vi "gfitsio-write-image-vi-data.vi"(7 "requested data":T1(ring)=enum."diagram, panel, .vi file", 8 "error in (no error)":errorcluster, 9 "vi depth (1)":i32=1, 11 "gfits refnum":T2=refnum) -> (0 "error out":errorcluster, 3 "dup gfits refnum":T2)   [LabVIEW 2013]
uses:
  gfitsio-refnum.ctl
  cfitsio-bitpix.ctl
  gfitsio-write-image-subset-variant.vi
  gfitsio-write-image-subset-u8-1d.vi
  gfitsio.lvlib
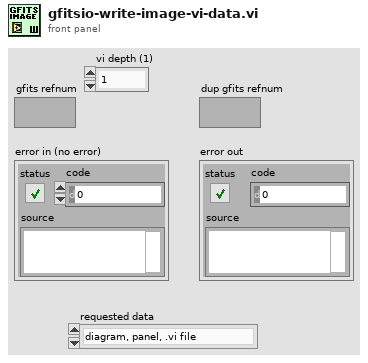
[diagram p1: front panel]
types:
  T1 = enum16{"diagram", "panel", ".vi file", "diagram, panel", "diagram, .vi file", "panel, .vi file", "diagram, panel, .vi file"}
  T2 = typedef "gfitsio.lvlib/gfitsio-refnum.ctl" = refnum<k1>
  T3 = typedef "gfitsio.lvlib/cfitsio-bitpix.ctl" = i32
  T4 = typedef "imagedata.ctl" = cluster{"image type":i32, "image depth":i32, "image":u8[], "mask":u8[], "colors":u32[], "Rectangle":cluster{"left":i16, "top":i16, "right":i16, "bottom":i16}}
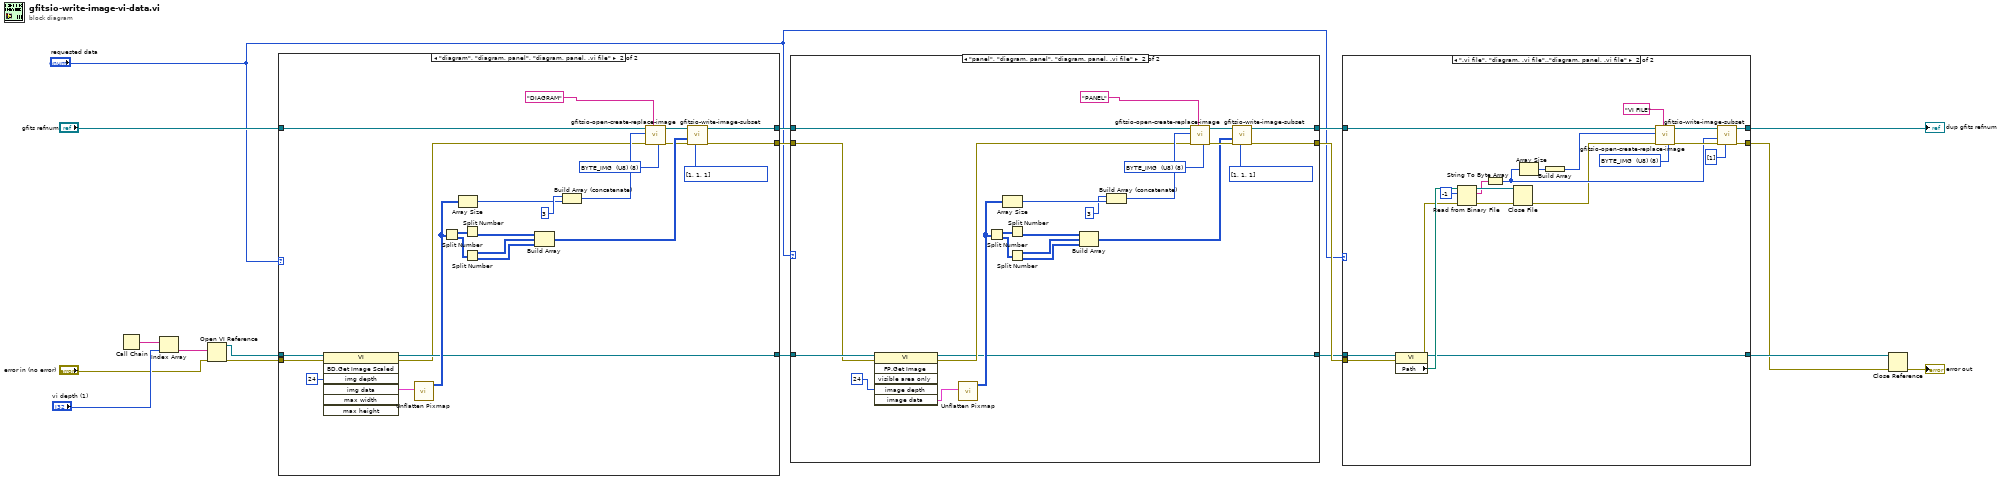
[diagram p0: block diagram]
diagram:
  n1 = Call Chain() -> (call chain=w17:string[])
  n2 = Index Array(array=w17, index="vi depth (1)") -> (element=w14:string)
  n3 = Open VI Reference(vi path=w14, error in (no error)="error in (no error)") -> (vi reference=w13:refnum<vi>, error out=w12:errorcluster)  [unwired: 4 in]
  n4 = case shown="\"diagram\", \"diagram, panel\", \"diagram, panel, .vi file\"" "requested data" {
    tunnel: "gfits refnum" -> [w19 w31]
    tunnel: w12 -> [w20 w28]
    tunnel: w13 -> [w21 w27]
    tunnel: [w19 w26] -> w10
    tunnel: [w21 w24] -> w9
    tunnel: [w20 w22] -> w8
    frame Default {
    }
    frame "diagram", "diagram, panel", "diagram, panel, .vi file" {
      w33 = T3 8 items=["<invalid type>"=0, "BYTE_IMG  (U8)"=8, "SHORT_IMG  (I16)"=16, "USHORT_IMG  (U16)"=20, "LONG_IMG  (I32)"=32, "ULONG_IMG  (U32)"=40, "FLOAT_IMG  (SGL)"=-32, "DOUBLE_IMG  (DBL)"=-64] ("image data type")
      n5 = invoke class="VI" method="BD.Get Image Scaled"(reference=w27, error in=w28, "img depth"=24 ("Image Depth")) -> (reference out=w24:refnum<vi>, error out=w23:errorcluster, "img data"=w29:T4)  [unwired: 4 in, 4 out]
      n6 = call <vilib>:"Unflatten Pixmap.vi"("image data"=w29) -> ("24-bit pixmap"=w36:u32[][])  [unwired: 4 in, 6 out]
      n7 = Split Number(x=w36) -> (hi(x)=w34:u16[][], lo(x)=w35:u16[][])
      n8 = Array Size(array=w36) -> (size(s)=w32:i32[])
      n9 = Split Number(x=w34) -> (lo(x)=w43:u8[][])  [unwired: 1 out]
      n10 = Split Number(x=w35) -> (hi(x)=w44:u8[][], lo(x)=w45:u8[][])
      n11 = Build Array(w43, w44, w45) -> (w42:u8[][][])
      n12 = Build Array (concatenate)(3, w32) -> (w40:i32[])
      n13 = call "gfitsio-open-create-replace-image.vi"("image data type"=w33, "hdu name (dialog if empty)"="DIAGRAM", "error in (no error)"=w23, "naxes"=w40, "gfits refnum"=w31) -> ("error out"=w37:errorcluster, "dup gfits refnum"=w38:T2)  [unwired: 4 in, 1 out]
      n14 = call-poly "gfitsio-write-image-subset.vi"("fpixel"=i32[] [1, 1, 1] ("size(s)"), "error in (no error)"=w37, "data"=w42, "gfits refnum"=w38) -> ("error out"=w22:errorcluster, "dup gfits refnum"=w26:T2)  [unwired: 6 in]
    }
  }
  n15 = case shown="\"panel\", \"diagram, panel\", \"diagram, panel, .vi file\"" "requested data" {
    tunnel: w10 -> [w48 w58]
    tunnel: w9 -> [w46 w56]
    tunnel: w8 -> [w47 w55]
    tunnel: [w47 w53] -> w7
    tunnel: [w46 w52] -> w6
    tunnel: [w48 w51] -> w2
    frame Default {
    }
    frame "panel", "diagram, panel", "diagram, panel, .vi file" {
      w71 = T3 8 items=["<invalid type>"=0, "BYTE_IMG  (U8)"=8, "SHORT_IMG  (I16)"=16, "USHORT_IMG  (U16)"=20, "LONG_IMG  (I32)"=32, "ULONG_IMG  (U32)"=40, "FLOAT_IMG  (SGL)"=-32, "DOUBLE_IMG  (DBL)"=-64] ("image data type")
      n16 = invoke class="VI" method="FP.Get Image"(reference=w56, error in=w55, "image depth"=24 ("Image Depth")) -> (reference out=w52:refnum<vi>, error out=w54:errorcluster, "image data"=w49:T4)  [unwired: 3 in, 3 out]
      n17 = call <vilib>:"Unflatten Pixmap.vi"("image data"=w49) -> ("24-bit pixmap"=w68:u32[][])  [unwired: 4 in, 6 out]
      n18 = Split Number(x=w68) -> (hi(x)=w70:u16[][], lo(x)=w69:u16[][])
      n19 = Array Size(array=w68) -> (size(s)=w72:i32[])
      n20 = Split Number(x=w70) -> (lo(x)=w61:u8[][])  [unwired: 1 out]
      n21 = Split Number(x=w69) -> (hi(x)=w60:u8[][], lo(x)=w59:u8[][])
      n22 = Build Array(w61, w60, w59) -> (w62:u8[][][])
      n23 = Build Array (concatenate)(3, w72) -> (w64:i32[])
      n24 = call "gfitsio-open-create-replace-image.vi"("image data type"=w71, "hdu name (dialog if empty)"="PANEL", "error in (no error)"=w54, "naxes"=w64, "gfits refnum"=w58) -> ("error out"=w67:errorcluster, "dup gfits refnum"=w66:T2)  [unwired: 4 in, 1 out]
      n25 = call-poly "gfitsio-write-image-subset.vi"("fpixel"=i32[] [1, 1, 1] ("size(s)"), "error in (no error)"=w67, "data"=w62, "gfits refnum"=w66) -> ("error out"=w53:errorcluster, "dup gfits refnum"=w51:T2)  [unwired: 6 in]
    }
  }
  n26 = case shown="\".vi file\", \"diagram, .vi file\"..\"diagram, panel, .vi file\"" "requested data" {
    tunnel: [w75 w83] -> w11
    tunnel: w7 -> [w74 w82]
    tunnel: w6 -> [w73 w79]
    tunnel: [w73 w78] -> w5
    tunnel: [w74 w77] -> w4
    tunnel: w2 -> [w75 w76]
    frame Default {
    }
    frame ".vi file", "diagram, .vi file".."diagram, panel, .vi file" {
      w87 = T3 8 items=["<invalid type>"=0, "BYTE_IMG  (U8)"=8, "SHORT_IMG  (I16)"=16, "USHORT_IMG  (U16)"=20, "LONG_IMG  (I32)"=32, "ULONG_IMG  (U32)"=40, "FLOAT_IMG  (SGL)"=-32, "DOUBLE_IMG  (DBL)"=-64] ("image data type")
      n27 = property class="VI"(reference=w79, error in=w82) -> (reference out=w78:refnum<vi>, error out=w81:errorcluster, "Path"=w85:path)
      n28 = Read from Binary File(8:w81, 10:-1 ("count (1)"), 11:w85) -> (0:w96:errorcluster, 2:w94:string, 3:w95:refnum<file>)  [unwired: 3 in, 1 out]
      n29 = String To Byte Array(string=w94) -> (unsigned byte array=w90:u8[])
      n30 = Close File(refnum=w95, error in=w96) -> (error out=w80:errorcluster)  [unwired: 1 out]
      n31 = Array Size(array=w90) -> (size(s)=w89:i32)
      n32 = Build Array(w89) -> (w88:i32[])
      n33 = call "gfitsio-open-create-replace-image.vi"("image data type"=w87, "hdu name (dialog if empty)"="VI FILE", "error in (no error)"=w80, "naxes"=w88, "gfits refnum"=w76) -> ("error out"=w92:errorcluster, "dup gfits refnum"=w93:T2)  [unwired: 4 in, 1 out]
      n34 = call-poly "gfitsio-write-image-subset.vi"("fpixel"=i32[] [1], "error in (no error)"=w92, "data"=w90, "gfits refnum"=w93) -> ("error out"=w77:errorcluster, "dup gfits refnum"=w83:T2)  [unwired: 6 in]
    }
  }
  "dup gfits refnum" <- w11
  n35 = Close Reference(reference=w5, error in (no error)=w4) -> (error out=→"error out":errorcluster)
